vi "Initialise devices.vi"() -> (5 "DLL Version":string, 6 "Device handles":u32[](array[numeric]), 8 "DLL error":errorcluster, 9 "Device initialisation errors":errorcluster[](array[cluster]), 10 "Device detection error":errorcluster)   [LabVIEW 2014]
uses:
  Commands.ctl
  Coherent global.vi
  Program Files (x86)/Coherent/HOPS/CohrHOPS.dll
panel:
  out "Laser comms. error":errorcluster[](array[cluster])
  out "Get lasers serial num. error":errorcluster
  out "Number of connected devices":u32
  # "PN 04/11/2014"
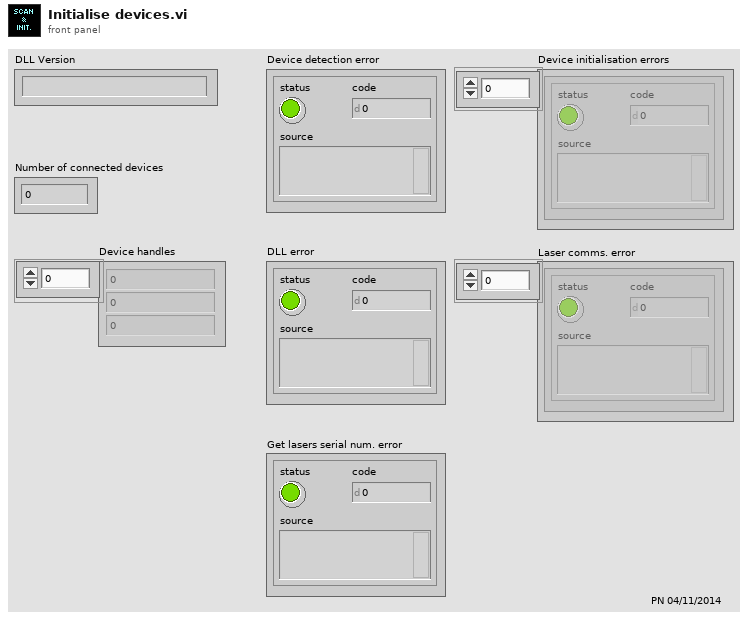
[diagram p1: front panel]
types:
  T1 = typedef "Commands.ctl" = u8
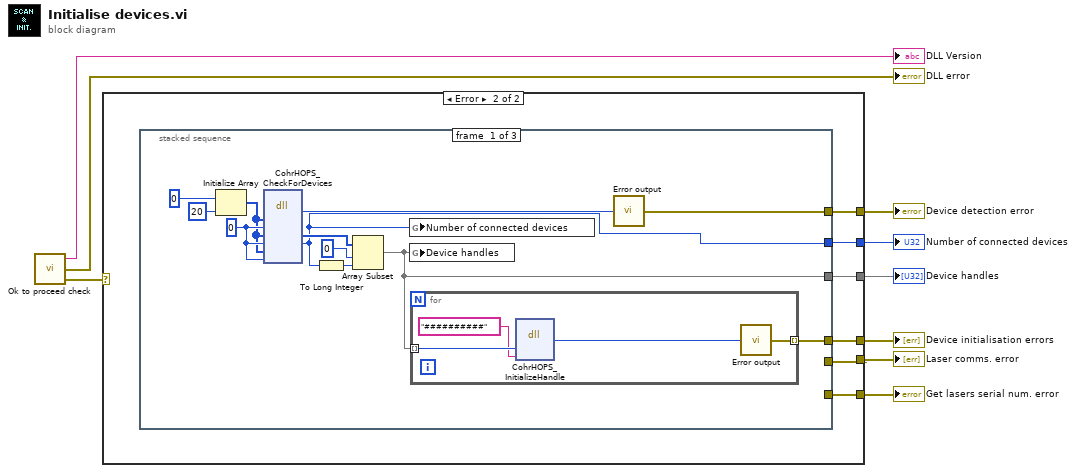
[diagram p0: block diagram]
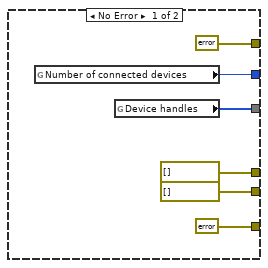
[diagram p2: hidden frame]
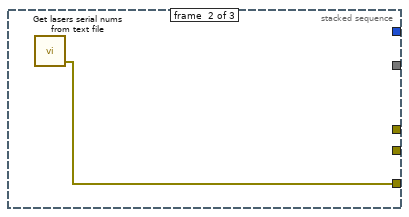
[diagram p3: hidden frame]
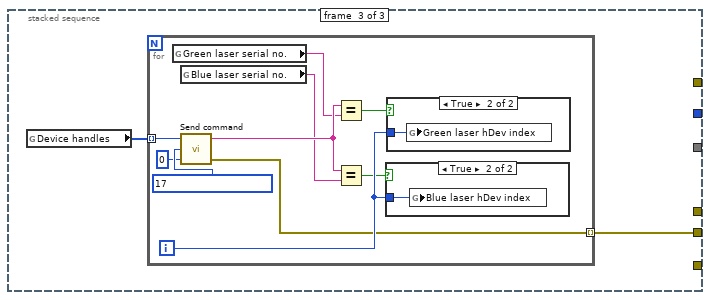
[diagram p4: hidden frame]
diagram:
  n1 = call "Ok to proceed check.vi"() -> ("Ok to proceed (error)"=w2:errorcluster, "DLL error"=→"DLL error":errorcluster, "DLL version"=→"DLL Version":string)  [unwired: 3 in]
  n2 = case shown="Error" w2 {
    tunnel: [w12 w21] -> w9
    tunnel: [errorcluster {"status"=FALSE, "code"=0, "source"=""} ("Error Out") w20] -> w8
    tunnel: [errorcluster[] [] w19] -> w7
    tunnel: [w13 w18] -> w6
    tunnel: [errorcluster {"status"=FALSE, "code"=0, "source"=""} ("Error") w17] -> w5
    tunnel: [errorcluster[] [] w16] -> w4
    frame No Error {
      n3 = global read "Coherent global.vi" "Number of connected devices"() -> (w13:u32)
      n4 = global read "Coherent global.vi" "Device handles"() -> (w12:u32[])
    }
    frame Error {
      n5 = stacked-sequence {
        tunnel: [w26 _ _] -> w21
        tunnel: [w25 _ _] -> w20
        tunnel: [w24 _ _] -> w19
        tunnel: [w22 _ _] -> w18
        tunnel: [_ w38 _] -> w17
        tunnel: [_ _ w39] -> w16
        frame #0 {
          w33 = u32 0 ("Input Value")
          n6 = Initialize Array(u32 0 ("Input Value"), 20 ("dimension size")) -> (w30:u32[])
          n7 = dll-call lib="C:/Program Files (x86)/Coherent/HOPS/CohrHOPS.dll" fn="CohrHOPS_CheckForDevices"("devicesConnected"=w30, "numberOfDevicesConnected"=w33, "devicesAdded"=w30, "numberOfDevicesAdded"=w33, "devicesRemoved"=w30, "numberOfDevicesRemoved"=w33) -> ("return value"=w27:i32, "devicesAdded"=w23:u32[], "numberOfDevicesAdded"=w22:u32)  [unwired: 7 in, 2 out]
          n8 = To Long Integer(number=w22) -> (32bit integer=w29:i32)
          n9 = Array Subset(array=w23, index=0, length=w29) -> (w26:u32[])
          n10 = global write "Coherent global.vi" "Number of connected devices"(w22) -> ()
          n11 = global write "Coherent global.vi" "Device handles"(w26) -> ()
          n12 = for {
            tunnel: w26 -> [w37] mode=indexing
            tunnel: [w35] -> w24 mode=indexing
            n13 = dll-call lib="C:/Program Files (x86)/Coherent/HOPS/CohrHOPS.dll" fn="CohrHOPS_InitializeHandle"("handle"=w37, "headType"="##########") -> ("return value"=w36:i32)  [unwired: 5 in, 2 out]
            n14 = call "Error output.vi"("I32 err code"=w36) -> ("Error Out"=w35:errorcluster)
          }
          n15 = call "Error output.vi"("I32 err code"=w27) -> ("Error Out"=w25:errorcluster)
        }
        frame #1 {
          n16 = call "Get lasers serial nums from text file.vi"() -> ("Error"=w38:errorcluster)  [unwired: 2 in, 2 out]
        }
        frame #2 {
          n17 = global read "Coherent global.vi" "Device handles"() -> (w40:u32[])
          n18 = for {
            tunnel: w40 -> [w49] mode=indexing
            tunnel: [w47] -> w39 mode=indexing
            i -> [w50]
            n19 = global read "Coherent global.vi" "Green laser serial no."() -> (w44:string)
            n20 = global read "Coherent global.vi" "Blue laser serial no."() -> (w45:string)
            n21 = call "Send command.vi"("Value"=u16 0, "Command"=T1 17, "Device handle"=w49) -> ("Error"=w47:errorcluster, "response"=w46:string)  [unwired: 1 out]
            n22 = Equal?(x=w46, y=w44) -> (x = y?=w43:bool)
            n23 = Equal?(x=w46, y=w45) -> (x = y?=w42:bool)
            n24 = case shown="True" w42 {
              tunnel: w50 -> [_ w52]
              frame False {
              }
              frame True {
                n25 = global write "Coherent global.vi" "Blue laser hDev index"(w52) -> ()
              }
            }
            n26 = case shown="True" w43 {
              tunnel: w50 -> [_ w51]
              frame False {
              }
              frame True {
                n27 = global write "Coherent global.vi" "Green laser hDev index"(w51) -> ()
              }
            }
          }
        }
      }
    }
  }
  "Device handles" <- w9
  "Device detection error" <- w8
  "Device initialisation errors" <- w7
  "Number of connected devices" <- w6
  "Get lasers serial num. error" <- w5
  "Laser comms. error" <- w4
